vi "AuMT8852B EDR Maximum Input Power Results.vi"(8 "error in (no error)":errorcluster, 11 "VISA session":refnum<visa-resource-name>) -> (0 "error out":errorcluster, 2 "error code":i32, 3 "VISA session out":refnum<visa-resource-name>, 4 "Results":T1 {"3MBs Overall BER" format="%.2e"; "2MBs Overall BER" format="%.2e"})   [LabVIEW 2017]
doc: "Anritsu MT8852B Bluetooth Tester\n\nReturns the summary results of the EDR Sensitivity test.\n\nOUTPUT\nResults - measurements made during the test."
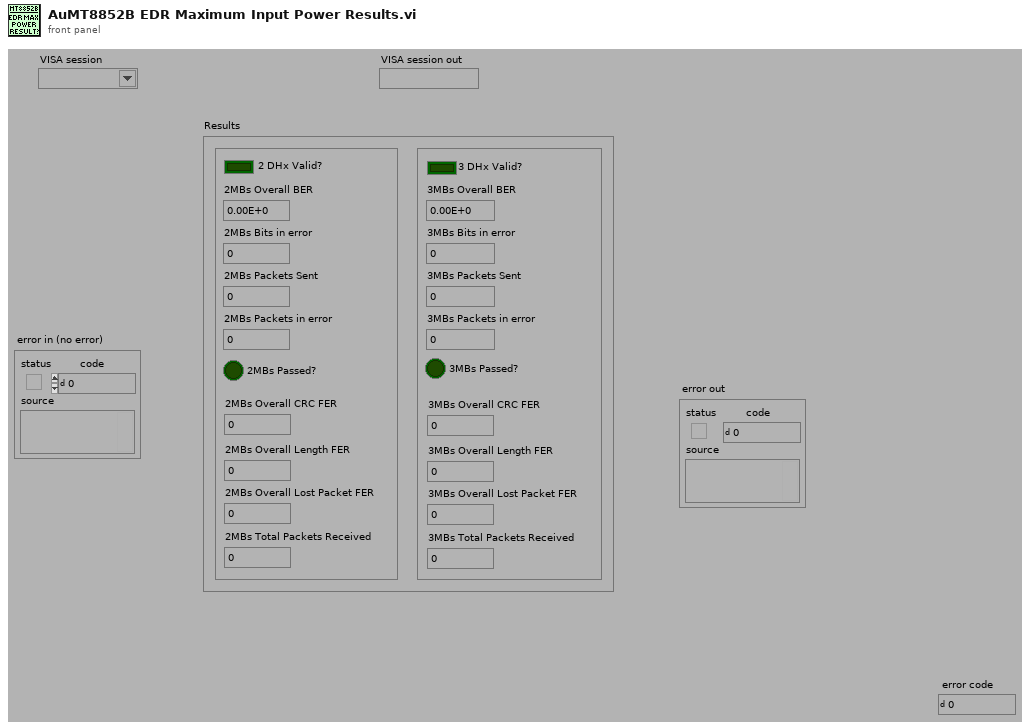
[diagram p1: front panel]
types:
  T1 = cluster{"2 DHx Valid?":bool, "2MBs Overall BER":dbl, "2MBs Bits in error":u32, "2MBs Packets Sent":u32, "2MBs Packets in error":u32, "3 DHx Valid?":bool, "3MBs Overall BER":dbl, "3MBs Bits in error":u32, "3MBs Packets Sent":u32, "3MBs Passed?":bool, "3MBs Packets in error":u32, "2MBs Overall CRC FER":u32, "2MBs Overall Length FER":u32, "2MBs Overall Lost Packet FER":u32, "3MBs Overall CRC FER":u32, "3MBs Overall Length FER":u32, "3MBs Overall Lost Packet FER":u32, "2MBs Total Packets Received":u32, "3MBs Total Packets Received":u32, "2MBs Passed?":bool}
  T2 = enum16{"Simulate", "Range check", "Cache", "Query instrument status"}
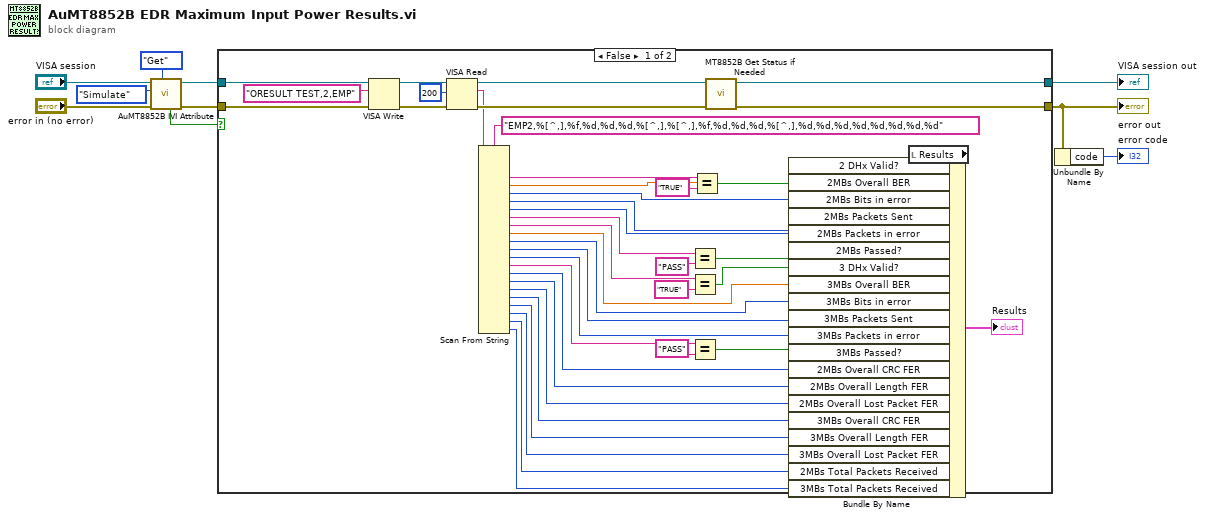
[diagram p0: block diagram]
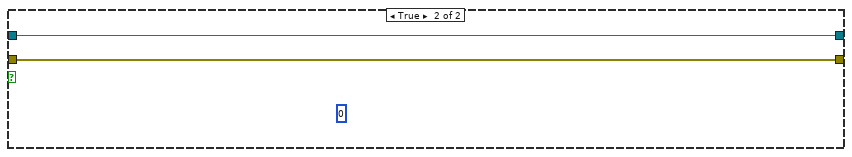
[diagram p2: hidden frame]
diagram:
  n1 = call <instrlib>:"AuMT8852B IVI Attribute.vi"("Set/Get (Set)"=enum16{"Set", "Get"}."Get", "error in (no error)"="error in (no error)", "Flag (Simulate)"=T2."Simulate", "VISA session"="VISA session") -> ("error out"=w7:errorcluster, "VISA session out"=w9:refnum<visa-resource-name>, "Value out"=w3:bool)  [unwired: 5 in]
  n2 = case shown="False" w3 {
    tunnel: [w44 w54] -> w10
    tunnel: [w43 w53] -> w1
    tunnel: w9 -> [w51 w54]
    tunnel: w7 -> [w50 w53]
    frame False {
      n3 = VISA Write(VISA resource name=w51, write buffer="ORESULT TEST,2,EMP" ("write buffer (\"\")"), error in (no error)=w50) -> (VISA resource name out=w49:refnum<visa-resource-name>, error out=w48:errorcluster)  [unwired: 1 out]
      n4 = VISA Read(VISA resource name=w49, byte count=u32 200 ("byte count (0)"), error in (no error)=w48) -> (VISA resource name out=w42:refnum<visa-resource-name>, read buffer=w40:string, error out=w41:errorcluster)  [unwired: 1 out]
      n5 = Scan From String(format string="EMP2,%[^,],%f,%d,%d,%d,%[^,],%[^,],%f,%d,%d,%d,%[^,],%d,%d,%d,%d,%d,%d,%d,%d" ("Format String"), input string=w40) -> (output 1=w39:string, output 2=w35:dbl, output 3=w34:i32, output 4=w33:i32, output 5=w31:i32, output 6=w30:string, output 7=w26:string, output 8=w25:dbl, output 9=w24:i32, output 10=w23:i32, output 11=w22:i32, output 12=w21:string, output 13=w18:i32, output 14=w17:i32, output 15=w16:i32, output 16=w15:i32, output 17=w14:i32, output 18=w13:i32, output 19=w12:i32, output 20=w11:i32)  [unwired: 22 in, 3 out]
      n6 = Equal?(x=w30, y="PASS") -> (x = y?=w29:bool)
      n7 = Equal?(x=w26, y="TRUE") -> (x = y?=w27:bool)
      n8 = Equal?(x=w21, y="PASS") -> (x = y?=w20:bool)
      n9 = Equal?(x=w39, y="TRUE") -> (x = y?=w36:bool)
      n10 = call <instrlib>:"MT8852B Get Status if Needed.vi"("error in (no error)"=w41, "VISA session"=w42) -> ("error out"=w43:errorcluster, "VISA session out"=w44:refnum<visa-resource-name>)  [unwired: 8 in]
      n11 = local read "Results"() -> (w37:T1)
      n12 = Bundle By Name(cluster=w37, "2 DHx Valid?"=w36, "2MBs Overall BER"=w35, "2MBs Bits in error"=w34, "2MBs Packets Sent"=w33, "2MBs Packets in error"=w31, "2MBs Passed?"=w29, "3 DHx Valid?"=w27, "3MBs Overall BER"=w25, "3MBs Bits in error"=w24, "3MBs Packets Sent"=w23, "3MBs Packets in error"=w22, "3MBs Passed?"=w20, "2MBs Overall CRC FER"=w18, "2MBs Overall Length FER"=w17, "2MBs Overall Lost Packet FER"=w16, "3MBs Overall CRC FER"=w15, "3MBs Overall Length FER"=w14, "3MBs Overall Lost Packet FER"=w13, "2MBs Total Packets Received"=w12, "3MBs Total Packets Received"=w11) -> (→"Results":T1)
    }
    frame True {
      (unwired) u8 0
    }
  }
  "error out" <- w1
  "VISA session out" <- w10
  n13 = Unbundle By Name(w1) -> ("code"=→"error code":i32)
